vi "ADC SNR_new.vi"(8 "error in (no error)":errorcluster, 9 "Sequence parameters":string[][](array[string])=[["Min limit", "Max limit", "Register sheet file", "Register Sheet"], ["", "", "CC2600.xls", "TX_BLE;Trim"], ["Reg write (addr;value)", "Operating frequency [Hz]", "", ""], ["NA", "2.44G", "", ""]], 10 "Run type":i32, 11 "Method parameters":T4={"Dev"={"Do not disturb DUT"=FALSE, "XOSC"=32000000.0, "Board type"="", "EM"="", "Configure tempboard"=TRUE, "Device specific info"=[], "Generic Object"=refnum}, "Method"={"Run type"=1, "Test name"="Current LPM2 4", "Comment"="", "Results folder"="", "AFC"=enum."Off", "Method name"="Current LPM2 4", "Method results"={"Excel brief report"=FALSE, "Spotfire report"=FALSE, "Starfish report"=FALSE}, "Operator"="", "Reference time"=timestamp(0 s since 1904-01-01), "AFC delay"=0.0, "Initialization"=enum."Enabled", "MD5 Sum"="", "HW addon board"=enum."None", "AFC Regsheet"="", "AFC Regfile"=path "", "dummy"=0.0}, "Inst"={"Instr"={"PS1"={"Name"="", "GPIB address"="", "VISA session"=""}, "PS2"={"Name"="", "GPIB address"="", "VISA session"=""}, "TC1"={"Name"="", "GPIB address"="", "VISA session"=""}, "TC2"={"Name"="", "GPIB address"="", "VISA session"=""}, "SA1"={"Name"="", "GPIB address"="", "VISA session"=""}, "SA2"={"Name"="", "GPIB address"="", "VISA session"=""}, "SG1"={"Name"="", "GPIB address"="", "VISA session"=""}, "SG2"={"Name"="", "GPIB address"="", "VISA session"=""}, "SG3"={"Name"="", "GPIB address"="", "VISA session"=""}, "MI1"={"Name"="", "GPIB address"="", "VISA session"=""}, "MI2"={"Name"="", "GPIB address"="", "VISA session"=""}, "SW SA"={"Name"="", "Controller addr"=""}, "SW SG"={"Name"="", "Controller addr"=""}, "MI3"={"Name"="", "GPIB address"="", "VISA session"=""}}, "Switchbox"={"RF Path"=0, "Cal compensation"=enum."TX", "Switchbox gain mode"="", "State"=enum."TX"}, "Instr to control (i.e. SA1)"="Default", "Intrument info string"=""}, "Sequence parameters"=[["Weight", "Min Limit", "Max Limit", "Register Sheet", "", "", "", "", "", "", "", "", ""], ["Vital", "", "1", "LPM2", "", "", "", "", "", "", "", "", ""], ["Resolution", "Reg write (addr;value)", "Chip mode", "Range", "", "", "", "", "", "", "", "", ""], ["u", "NA", "", "auto", "", "", "", "", "", "", "", "", ""]], "Cond"={"Temp logged"=25.0, "VDD1_PS1_6V"=-999.0, "VDD2_PS1_25V"=-999.0, "VDD4_PS2_25V"=-999.0, "VDD3_PS2_6V"=-999.0}, "Meas config"={"X-axis inner loop index"=32000000, "Y-axis outer loop index"=32000000, "X-axis"=[], "Y-axis"=[], "X-axis array req size"=32000000, "Y-axis array req size"=32000000, "Param description"=[], "Use meas clust for reporting"=FALSE, "Parameter index (page)"=0, "X-axis name"="", "Y-axis name"=""}} {"Cond"."VDD3_PS2_6V" format="%.3f"; "Cond"."VDD4_PS2_25V" format="%.3f"; "Cond"."VDD2_PS1_25V" format="%.3f"; "Cond"."VDD1_PS1_6V" format="%.3f"; "Method"."dummy" format="%.1p"; "Method"."AFC delay" format="%.1p"; "Dev"."XOSC" format="%.3p"}) -> (0 "error out":errorcluster, 1 "End method error":T2, 2 "Short Results":string[](array[string])=["0.00", "0.00", "0.00", "0.00"], 3 "Result summary":string[][](array[string])=[["Critical", "Output Power@2405 MHz", "-3", "4", "dBm"], ["Critical", "Output Power@2410 MHz", "-3", "4", "dBm"]])   [LabVIEW 2019]
doc: "[AutoDocStart]Performs crystal accuracy measurements. Measures the offset from ideal frequency. Primarily used for tuning XOSC capacitors and verifying XOSC trims.\n\nSweeping parameters: operating frequency, OSC override value and VDDR level\n\nResults: Offset frequency in ppm[AutoDocEnd]"
uses:
  User Lib/Utilities/Cluster definitions/DUT VDD1.ctl
  User Lib/Utilities/Cluster definitions/DUT VDD2.ctl
  User Lib/Utilities/Cluster definitions/DUT VDD3.ctl
  User Lib/Utilities/Cluster definitions/DUT VDD4.ctl
  User Lib/Utilities/Cluster definitions/DUT vdd control.ctl
  User Lib/Generic chip methods/Classes/Generic_EM/Chameleon/Loki/Loki.lvclass
  User Lib/Generic chip methods/Classes/Generic_EM/Generic_EM/Generic_EM.lvclass
  User Lib/Utilities/Cluster definitions/Instr clust.ctl
  User Lib/Utilities/Cluster definitions/Method input.ctl
  User Lib/Utilities/Controls/Automatic Frequency Compensation types.ctl
  User Lib/Utilities/Controls/Method Reports.ctl
  User Lib/Utilities/Cluster definitions/End method error cluster.ctl
  User Lib/Utilities/Cluster definitions/Device specific info.ctl
  User Lib/Utilities/Cluster definitions/Method Initialization.ctl
  User Lib/Utilities/Switchbox control/SwitchBox_State._ENUMctl.ctl
  User Lib/Utilities/Controls/HW addon boards.ctl
panel:
  in  "Tab Control":T1(tab)
  out "Dynamic Parameters":T3={"SNR"=nan, "SNRD"=nan, "THD"=nan, "ENOB (SNRD)"=nan, "SFDR"=nan, "ENOB (SNR)"=nan, "Noise Power"=nan, "Signal power"=nan} {"Signal power" format="%.6f"; "Noise Power" format="%.2f"; "ENOB (SNR)" format="%.2f"; "SFDR" format="%.2f"; "ENOB (SNRD)" format="%.2f"; "THD" format="%.2f"; "SNRD" format="%.2f"; "SNR" format="%.2f"}
  out "ADC samples":u32[](array[numeric])
  out "Output Response [All DUTs]":u32[][](array[numeric])
  out "SNR":dbl
  out "Noise Power":dbl
  out "Signal power":dbl
  out "ENOB (SNR)":dbl
  out "detected Throughput":dbl=200065.4236150998
  # "°C"
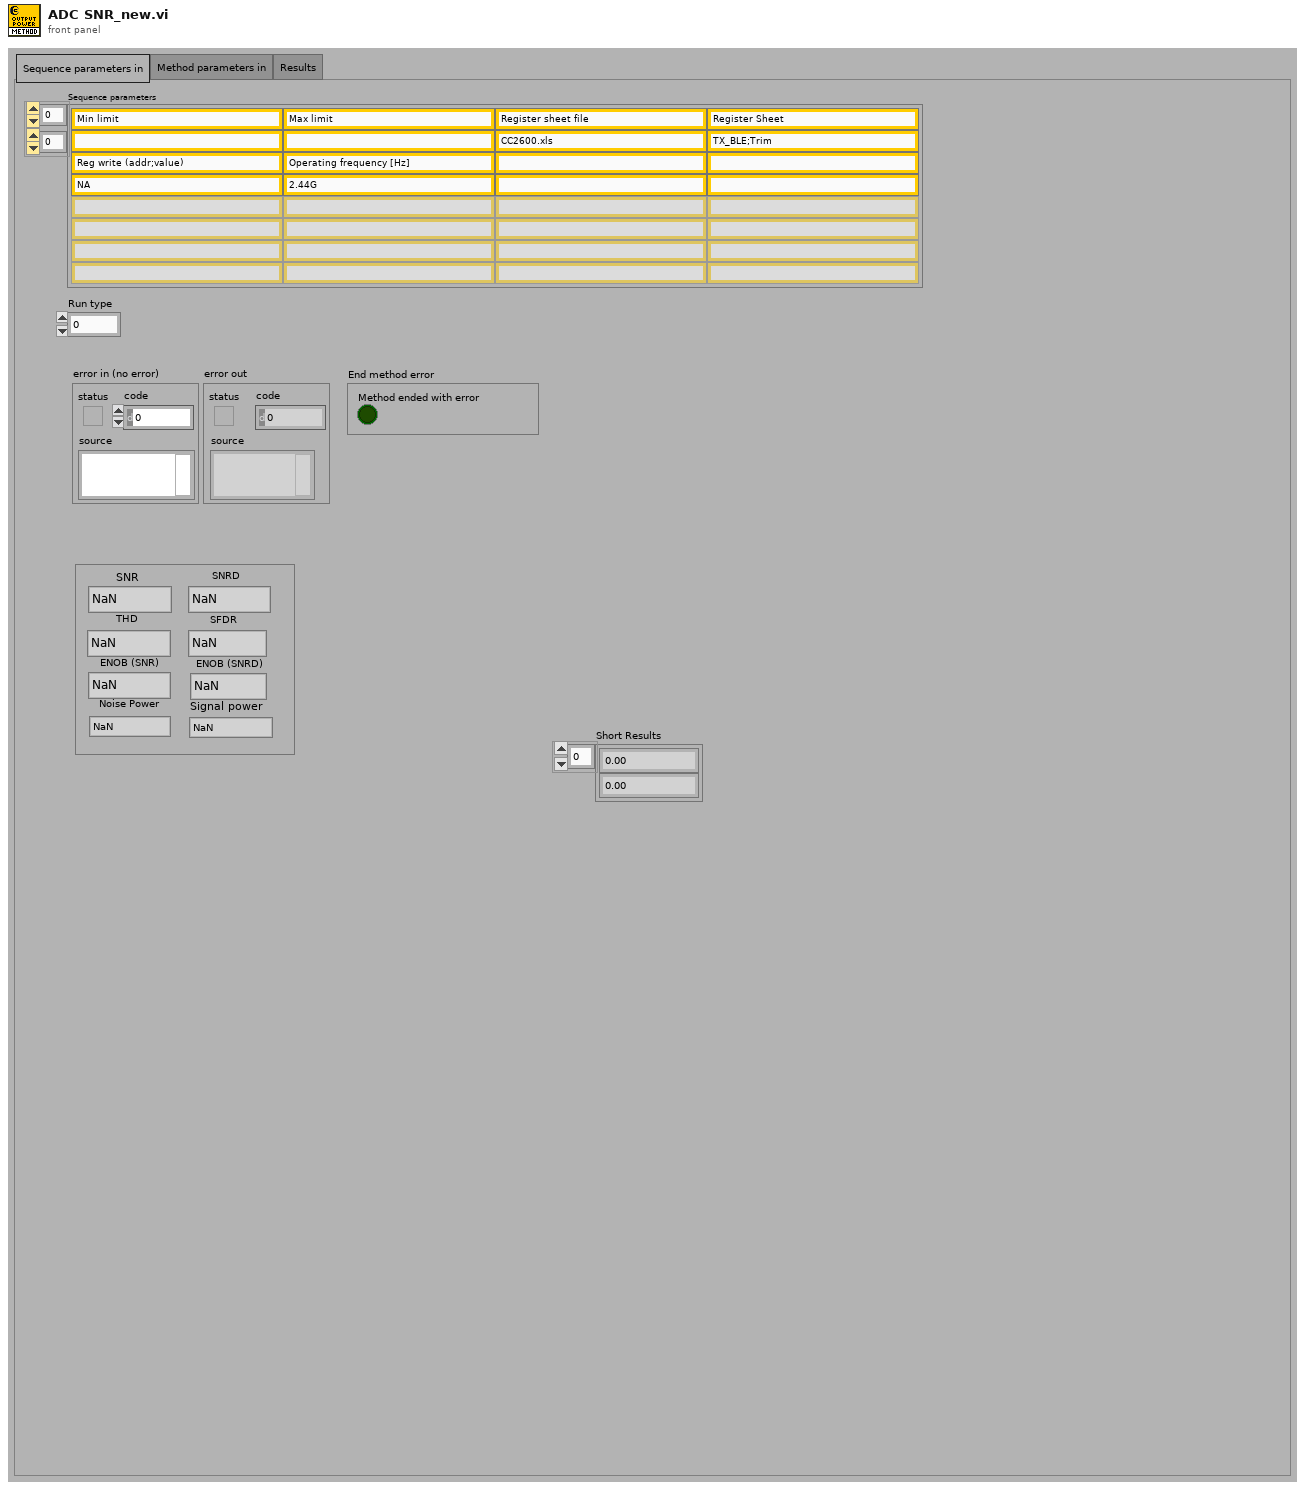
[diagram p1: front panel]
types:
  T1 = enum32{"Sequence parameters in", "Method parameters in", "Results"}
  T2 = typedef "End method error cluster.ctl" = cluster{"Method ended with error":bool}
  T3 = cluster{"SNR":dbl, "SNRD":dbl, "THD":dbl, "ENOB (SNRD)":dbl, "SFDR":dbl, "ENOB (SNR)":dbl, "Noise Power":dbl, "Signal power":dbl}
  T4 = typedef "Method input.ctl" = cluster{"Dev":cluster{"Do not disturb DUT":bool, "XOSC":dbl, "Board type":string, "EM":string, "Configure tempboard":bool, "Device specific info":T5[], "Generic Object":refnum<class>}, "Method":cluster{"Run type":i32, "Test name":string, "Comment":string, "Results folder":string, "AFC":T6, "Method name":string, "Method results":T7, "Operator":string, "Reference time":timestamp, "AFC delay":dbl, "Initialization":T8, "MD5 Sum":string, "HW addon board":T9, "AFC Regsheet":string, "AFC Regfile":path, "dummy":dbl}, "Inst":T10, "Sequence parameters":string[][], "Cond":cluster{"Temp logged":dbl, "VDD1_PS1_6V":dbl, "VDD2_PS1_25V":dbl, "VDD4_PS2_25V":dbl, "VDD3_PS2_6V":dbl}, "Meas config":cluster{"X-axis inner loop index":i32, "Y-axis outer loop index":i32, "X-axis":string[], "Y-axis":string[], "X-axis array req size":i32, "Y-axis array req size":i32, "Param description":string[][], "Use meas clust for reporting":bool, "Parameter index (page)":i32, "X-axis name":string, "Y-axis name":string}}
  T5 = typedef "Device specific info.ctl" = cluster{"EM number":u8, "IP address":string, "Enabled":bool, "Slot no":u8, "RF path":u8, "EM name":string, "Wafer info":string, "AFC frequency ppm":dbl, "Register writes":string[][], "Meas data":string[][][], "Device comment":string}
  T6 = typedef "Automatic Frequency Compensation types.ctl" = enum16{"Off", "Compensate Instrument frequency", "Compensate DUT frequency", "Predictive - Compensate Instrument frequency", "Predictive - Compensate DUT frequency", "Do not skip re-init - Compensate Instrument frequency", "Do not skip re-init - Compensate DUT frequency"}
  T7 = typedef "Method Reports.ctl" = cluster{"Excel brief report":bool, "Spotfire report":bool, "Starfish report":bool}
  T8 = typedef "Method Initialization.ctl" = enum16{"Enabled", "Skip Instr and Device Init", "Enabled with Separate Flash", "Set PS, Device Init and Skip Instr Init", "Skip Device Init"}
  T9 = typedef "HW addon boards.ctl" = enum16{"None", "Current meas 5EM", "Stresstest 10EM"}
  T10 = typedef "Instr clust.ctl" = cluster{"Instr":cluster{"PS1":cluster{"Name":string, "GPIB address":string, "VISA session":refnum<visa-resource-name>}, "PS2":cluster{"Name":string, "GPIB address":string, "VISA session":refnum<visa-resource-name>}, "TC1":cluster{"Name":string, "GPIB address":string, "VISA session":refnum<visa-resource-name>}, "TC2":cluster{"Name":string, "GPIB address":string, "VISA session":refnum<visa-resource-name>}, "SA1":cluster{"Name":string, "GPIB address":string, "VISA session":refnum<visa-resource-name>}, "SA2":cluster{"Name":string, "GPIB address":string, "VISA session":refnum<visa-resource-name>}, "SG1":cluster{"Name":string, "GPIB address":string, "VISA session":refnum<visa-resource-name>}, "SG2":cluster{"Name":string, "GPIB address":string, "VISA session":refnum<visa-resource-name>}, "SG3":cluster{"Name":string, "GPIB address":string, "VISA session":refnum<visa-resource-name>}, "MI1":cluster{"Name":string, "GPIB address":string, "VISA session":refnum<visa-resource-name>}, "MI2":cluster{"Name":string, "GPIB address":string, "VISA session":refnum<visa-resource-name>}, "SW SA":cluster{"Name":string, "Controller addr":string}, "SW SG":cluster{"Name":string, "Controller addr":string}, "MI3":cluster{"Name":string, "GPIB address":string, "VISA session":refnum<visa-resource-name>}}, "Switchbox":cluster{"RF Path":i32, "Cal compensation":enum16{"TX", "RX", "Interferer", "No compensation", "Interferer2"}, "Switchbox gain mode":string, "State":T11}, "Instr to control (i.e. SA1)":string, "Intrument info string":string}
  T11 = typedef "SwitchBox_State._ENUMctl.ctl" = enum16{"TX", "RX", "SP:TX", "SP:RX", "SW:TX", "SW:RX"}
  T12 = typedef "DUT vdd control.ctl" = cluster{"VDD4 config":T13, "VDD3 config":T14, "VDD2 config":T15, "VDD1 config":T16}
  T13 = typedef "DUT VDD4.ctl" = u16
  T14 = typedef "DUT VDD3.ctl" = u16
  T15 = typedef "DUT VDD2.ctl" = u16
  T16 = typedef "DUT VDD1.ctl" = u16
  T17 = cluster{"Path to Save plot":path, "Path to Raw Data plot":path}
  T18 = cluster{"Fundamental Frequency":dbl, "Sampling Frequncy":dbl, "No of Harmonics":u8, "Window":enum16{"None ", "Hanning", "Hamming", "Blackman-Harris", "Exact Blackman", "Blackman", "Flat Top", "4 Term B-Harris ", "7 Term B-Harris"}, "Blackman (fundamental power) bins)":dbl}
  T19 = cluster{"Save INL/DNL Plot(Ramp)":bool, "Save SNR Plot":bool, "Save INL/DNL Plot(Sine)":bool, "Save INL/DNL Raw Data(Ramp)":bool, "Save SNR Raw Data":bool, "Save INL/DNL Raw Data(Sine)":bool, "Save DC Raw data":bool, "Save  Raw Data(Sine)":bool}
  T20 = enum32{"NI Card Settings", "Memory Read Setting", "DC Capture", "ADC Ramp", "ADC Sine", "SNR", "Cap Calibration"}
  T21 = enum32{"Read from Memory", "Read .dat file", "NI Card Capture", "None"}
  T22 = typedef "TFW ResponseData.ctl" = cluster{"errorCode":u32, "executionTime":u32, "processedCmdWord":u32, "responsePar":u32[], "actionCode":u32, "cmdStatus":u16}
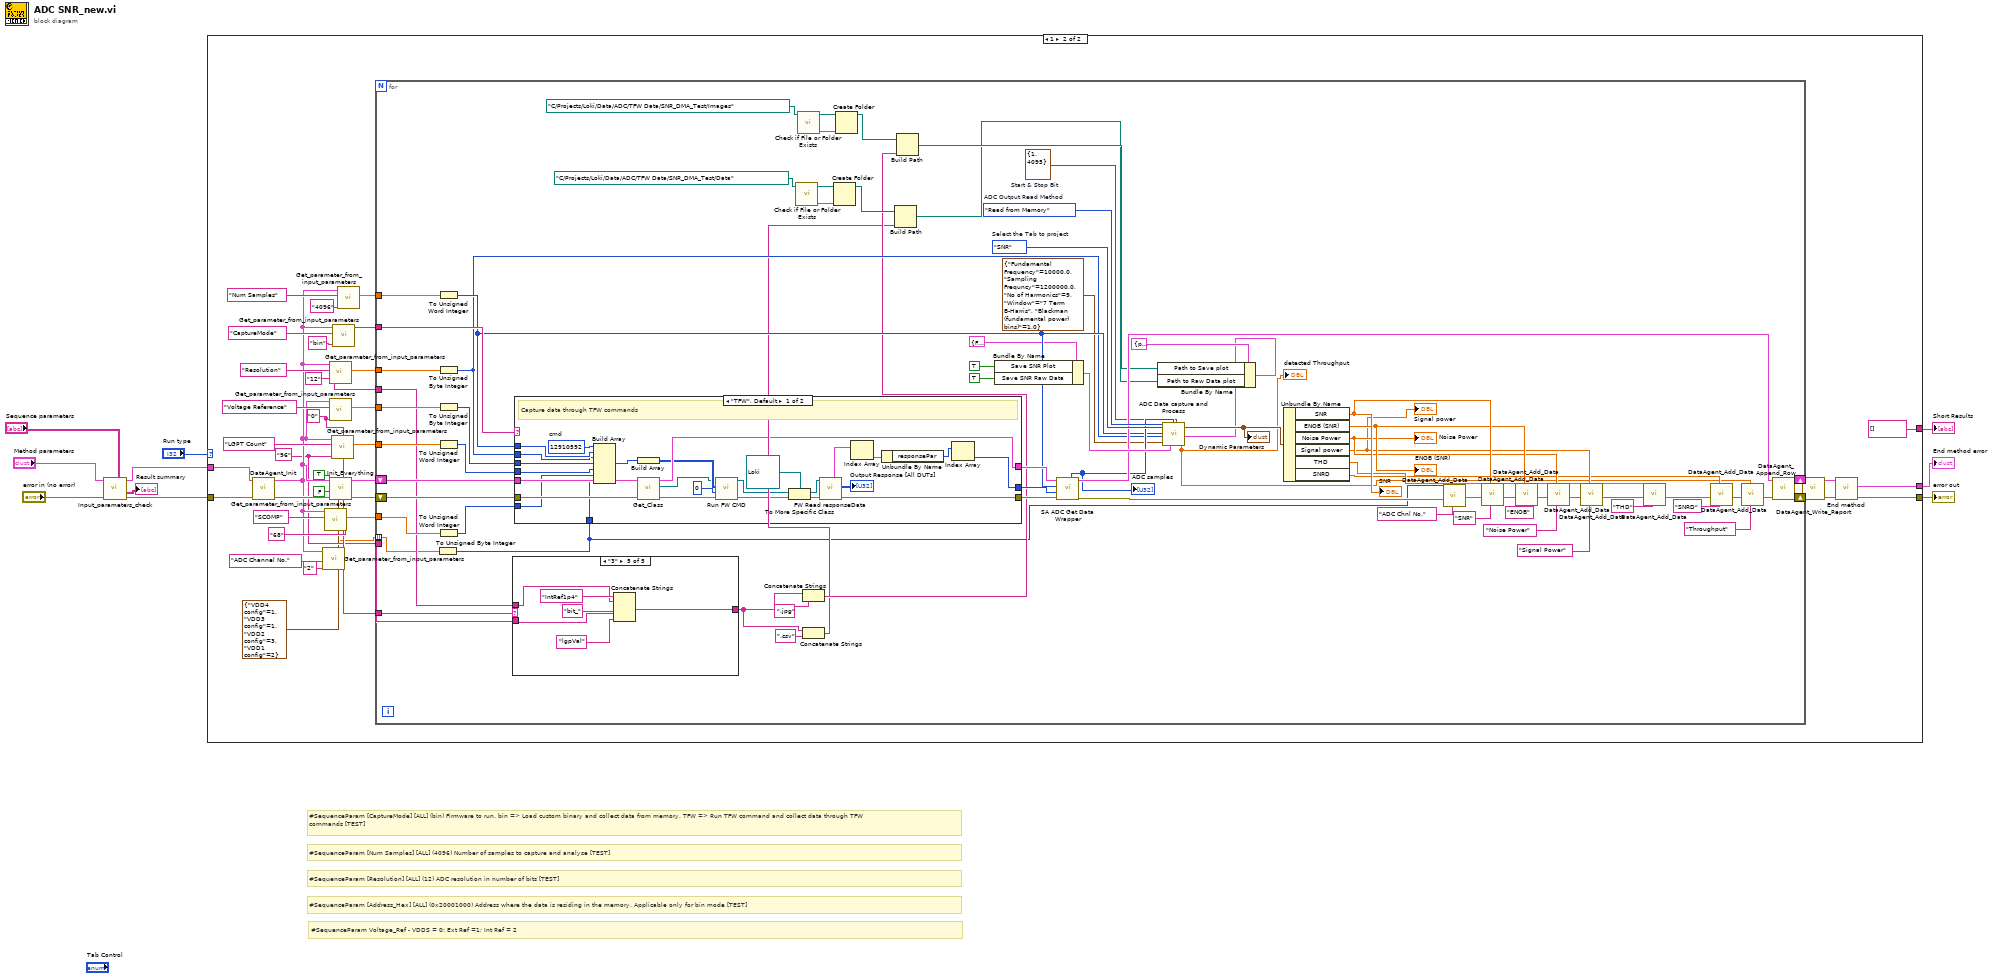
[diagram p0: block diagram]
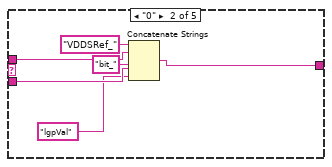
[diagram p4: hidden frame]
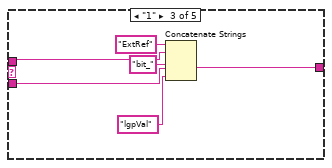
[diagram p5: hidden frame]
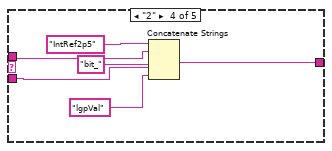
[diagram p6: hidden frame]
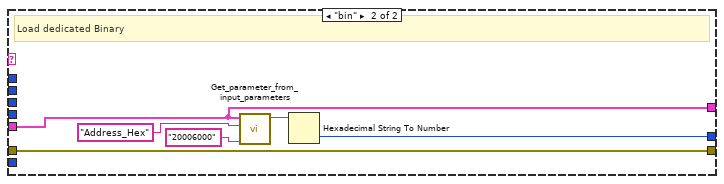
[diagram p7: hidden frame]
diagram:
  # "#SequenceParam Voltage_Ref - VDDS = 0; Ext Ref =1; Int Ref = 2"
  # "#SequenceParam [Num Samples] [ALL] (4096) Number of samples to capture and analyse [TEST]"
  # "#SequenceParam [CaptureMode] [ALL] (bin) Firmware to run. bin => Load custom binary and collect data from memory. TFW => Run TFW command and collect data through TFW commands [TEST]"
  # "#SequenceParam [Address_Hex] [ALL] (0x20001000) Address where the data is residing in the memory. Applicable only for bin mode [TEST]"
  # "#SequenceParam [Resolution] [ALL] (12) ADC resolution in number of bits [TEST]"
  n1 = call "Input_parameters_check.vi"("Sequence parameters"="Sequence parameters", "error in"="error in (no error)", "Method cluster in"="Method parameters") -> ("error out"=w9:errorcluster, "Result summary"=→"Result summary":string[][], "Method cluster out"=w5:T4)  [unwired: 6 in]
  n2 = case shown="1" "Run type" {
    tunnel: w9 -> [w11 w45]
    tunnel: [w11 w48] -> w10
    tunnel: w5 -> [_ w46]
    tunnel: [_ w47] -> w4
    tunnel: [_ string[] []] -> w1
    frame 0, Default {
      # "Run type 0 is only for formatting the result summary"
    }
    frame 1 {
      w15 = "96" ("Default value (used if not specified on Front Panel)")
      w19 = "0" ("Default value (used if not specified on Front Panel)")
      w18 = "12" ("Default value (used if not specified on Front Panel)")
      n3 = call "DataAgent_Init.vi"("error in (no error)"=w45, "Method cluster in"=w46) -> ("error out"=w44:errorcluster, "Method cluster out"=w17:T4)  [unwired: 8 in]
      n4 = call "Get_parameter_from_input_parameters.vi"("Default value (used if not specified on Front Panel)"="2", "Parameter name"="ADC Channel No.", "Method cluster (if input param empty)"=w17) -> ("value as DBL Array"=w13:dbl[])  [unwired: 2 in, 6 out]
      n5 = call "Get_parameter_from_input_parameters.vi"("Default value (used if not specified on Front Panel)"="68", "Parameter name"="SCOMP", "Method cluster (if input param empty)"=w17) -> ("value as DBL"=w20:dbl)  [unwired: 2 in, 6 out]
      n6 = call "Get_parameter_from_input_parameters.vi"("Default value (used if not specified on Front Panel)"=w18, "Parameter name"="Resolution" ("SA_ param name"), "Method cluster (if input param empty)"=w17) -> ("value as DBL"=w26:dbl)  [unwired: 2 in, 6 out]
      n7 = call "Get_parameter_from_input_parameters.vi"("Default value (used if not specified on Front Panel)"=w19, "Parameter name"="Voltage Reference", "Method cluster (if input param empty)"=w17) -> ("value as DBL"=w25:dbl)  [unwired: 2 in, 6 out]
      n8 = call "Init_Everything.vi"("VDD config"=T12 {"VDD4 config"=1, "VDD3 config"=1, "VDD2 config"=3, "VDD1 config"=2}, "error in"=w44, "Support current measurement?"=FALSE, "Override VDD Config"=TRUE, "Method cluster In"=w17) -> ("error out"=w41:errorcluster, "Method cluster out"=w40:T4)  [unwired: 3 in, 2 out]
      n9 = call "Get_parameter_from_input_parameters.vi"("Default value (used if not specified on Front Panel)"=w15, "Parameter name"="LGPT Count", "Method cluster (if input param empty)"=w17) -> ("value as DBL"=w21:dbl)  [unwired: 2 in, 6 out]
      n10 = call "Get_parameter_from_input_parameters.vi"("Default value (used if not specified on Front Panel)"="bin", "Parameter name"="CaptureMode" ("SA_ param name"), "Method cluster (if input param empty)"=w17) -> ("value as String"=w36:string)  [unwired: 2 in, 6 out]
      n11 = call "Get_parameter_from_input_parameters.vi"("Default value (used if not specified on Front Panel)"="4096", "Parameter name"="Num Samples" ("SA_ param name"), "Method cluster (if input param empty)"=w17) -> ("value as DBL"=w34:dbl)  [unwired: 2 in, 6 out]
      n12 = for {
        tunnel: w36 -> [w117]
        tunnel: w34 -> [w111]
        tunnel: w26 -> [w99]
        tunnel: w25 -> [w97]
        tunnel: w21 -> [w95]
        tunnel: w20 -> [w94]
        tunnel: w19 -> [w61]
        tunnel: w18 -> [w60]
        tunnel: w15 -> [w51]
        shift-right: [w108] -> w30
        shift-left: w41 -> [w123]
        shift-right: [w109] -> w31
        shift-left: w40 -> [w122]
        tunnel: w13 -> [w50] mode=indexing
        w100 = cluster{"Start":i32, "Stop":i32} {"Start"=1, "Stop"=4095}  # Start & Stop Bit
        w120 = T20."SNR"  # Select the Tab to project
        w121 = T21."Read from Memory"  # ADC Output Read Method
        n13 = To Unsigned Byte Integer(number=w50) -> (unsigned 8bit integer=w49:u8)
        n14 = To Unsigned Word Integer(number=w111) -> (unsigned 16bit integer=w110:u16)
        n15 = To Unsigned Byte Integer(number=w99) -> (unsigned 8bit integer=w98:u8)
        n16 = To Unsigned Byte Integer(number=w97) -> (unsigned 8bit integer=w96:u8)
        n17 = To Unsigned Word Integer(number=w95) -> (unsigned 16bit integer=w93:u16)
        n18 = To Unsigned Word Integer(number=w94) -> (unsigned 16bit integer=w92:u16)
        n19 = case shown="\"3\"" w61 {
          tunnel: w60 -> [w124 w129 w134 w140 w143]
          tunnel: w51 -> [_ w126 w132 w138 w144]
          tunnel: [w124 w127 w133 w139 w145] -> w58
          frame "False", Default {
          }
          frame "0" {
            n20 = Concatenate Strings("VDDSRef_" ("string"), w129, "bit_" ("string"), w126, "lgpVal" ("string")) -> (w127:string)
          }
          frame "1" {
            n21 = Concatenate Strings("ExtRef" ("string"), w134, "bit_" ("string"), w132, "lgpVal" ("string")) -> (w133:string)
          }
          frame "2" {
            n22 = Concatenate Strings("IntRef2p5" ("string"), w140, "bit_" ("string"), w138, "lgpVal" ("string")) -> (w139:string)
          }
          frame "3" {
            n23 = Concatenate Strings("IntRef1p4" ("string"), w143, "bit_" ("string"), w144, "lgpVal" ("string")) -> (w145:string)
          }
        }
        n24 = case shown="\"TFW\", Default" w117 {
          tunnel: [w174 w175] -> w114
          tunnel: [w167 w180] -> w113
          tunnel: w123 -> [w166 w180]
          tunnel: w122 -> [w173 w175]
          tunnel: [w154 w176] -> w112
          tunnel: w110 -> [w170 _]
          tunnel: w98 -> [w153 _]
          tunnel: w96 -> [w152 _]
          tunnel: w93 -> [w151 _]
          tunnel: w92 -> [w150 _]
          tunnel: w49 -> [w149 _]
          frame "TFW", Default {
            w171 = u32 12910592  # cmd
            # "Capture data through TFW commands"
            n25 = Build Array(w171, w170, w153, w152, w151, w150, w149) -> (w169:u32[])
            n26 = Build Array(w169) -> (w168:u32[][])
            n27 = call "Get_Class.vi"("error in (no error)"=w166, "Method cluster in"=w173) -> ("error out"=w164:errorcluster, "Class Out"=w163:refnum<class "Generic_EM.lvclass">, "Method cluster out"=w174:T4)  [unwired: 6 in, 1 out]
            n28 = call-dynamic "Run FW CMD.vi"("error in (no error)"=w164, "Handler"=u8 0, "cmdBuf"=w168, "Generic_EM in"=w163) -> ("error out"=w159:errorcluster, "Generic_EM out"=w162:refnum<class "Generic_EM.lvclass">)  [unwired: 6 in]
            n29 = To More Specific Class(target class=refnum<class "Loki.lvclass"> refnum ("Loki in"), reference=w162, error in=w159) -> (specific class reference=w160:refnum<class "Loki.lvclass">, error out=w158:errorcluster)
            n30 = call "FW Read responseData.vi"("error in (no error)"=w158, "Loki in"=w160) -> ("error out"=w167:errorcluster, "Output Response [All DUTs]"=→"Output Response [All DUTs]":u32[][], "Response"=w156:T22[])  [unwired: 6 in, 1 out]
            n31 = Index Array(array=w156) -> (element=w157:T22)  [unwired: 1 in]
            n32 = Unbundle By Name(w157) -> ("responsePar"=w155:u32[])
            n33 = Index Array(array=w155) -> (element=w154:u32)  [unwired: 1 in]
          }
          frame "bin" {
            # "Load dedicated Binary"
            n34 = call "Get_parameter_from_input_parameters.vi"("Default value (used if not specified on Front Panel)"="20006000", "Parameter name"="Address_Hex" ("SA_ param name"), "Method cluster (if input param empty)"=w175) -> ("value as String"=w179:string)  [unwired: 2 in, 6 out]
            n35 = Hexadecimal String To Number(string=w179) -> (number=w176:u32)  [unwired: 2 in, 1 out]
          }
        }
        n36 = call <vilib>:"Check if File or Folder Exists.vi"("path"=path "C:/Projects/Loki/Data/ADC/TFW Data/SNR_DMA_Test/Data" ("base path")) -> ("error out"=w66:errorcluster, "dup path"=w65:path)  [unwired: 8 in, 1 out]
        n37 = call <vilib>:"Check if File or Folder Exists.vi"("path"=path "C:/Projects/Loki/Data/ADC/TFW Data/SNR_DMA_Test/Images" ("base path")) -> ("error out"=w71:errorcluster, "dup path"=w70:path)  [unwired: 8 in, 1 out]
        n38 = Concatenate Strings(w58, ".jpg" ("string")) -> (w56:string)
        n39 = Concatenate Strings(w58, ".csv" ("string")) -> (w55:string)
        n40 = Create Folder(path (use dialog)=w65, error in=w66) -> (created path=w63:path)  [unwired: 1 in, 2 out]
        n41 = Create Folder(path (use dialog)=w70, error in=w71) -> (created path=w68:path)  [unwired: 1 in, 2 out]
        n42 = Build Path(base path=w63, name or relative path=w55) -> (appended path=w62:path)
        n43 = Build Path(base path=w68, name or relative path=w56) -> (appended path=w67:path)
        n44 = Bundle By Name(cluster=T19 {"Save INL/DNL Plot(Ramp)"=FALSE, "Save SNR Plot"=FALSE, "Save INL/DNL Plot(Sine)"=FALSE, "Save INL/DNL Raw Data(Ramp)"=FALSE, "Save SNR Raw Data"=FALSE, "Save INL/DNL Raw Data(Sine)"=FALSE, "Save DC Raw data"=FALSE, "Save  Raw Data(Sine)"=FALSE} ("Save data"), "Save SNR Plot"=TRUE, "Save SNR Raw Data"=TRUE) -> (w119:T19)
        n45 = call "SA ADC Get Data Wrapper.vi"("error in"=w113, "Data Address"=w112, "Num Samples"=w110, "Method cluster in"=w114) -> ("error out"=w54:errorcluster, "output cluster"=w116:T4, "ADC samples"=w115:u32[])  [unwired: 2 in, 3 out]
        "ADC samples" <- w115
        n46 = Bundle By Name(cluster=T17 {"Path to Save plot"=path "C:/Projects/Loki/Data/ADC/TFW Data/test.jpg", "Path to Raw Data plot"=path "C:/Projects/Loki/Data/ADC/TFW Data/test.csv"} ("path to save"), "Path to Save plot"=w67, "Path to Raw Data plot"=w62) -> (w90:T17)
        n47 = call "ADC Data capture and Process.vi"("ADC Output Read Method"=w121, "Select the Tab to project"=w120, "No.of samples(SNR)"=w110, "Resolution"=w98, "Inputs for Dyanmic para"=T18 {"Fundamental Frequency"=10000.0, "Sampling Frequncy"=1200000.0, "No of Harmonics"=9, "Window"=enum."7 Term B-Harris", "Blackman (fundamental power) bins)"=1.0}, "Save data"=w119, "Waveform"=w115, "Start & Stop Bit"=w100, "path to save"=w90) -> ("detected Throughput"=w73:dbl, "Dynamic Parameters"=w103:T3)  [unwired: 12 in, 5 out]
        "Dynamic Parameters" <- w103
        "detected Throughput" <- w73
        n48 = Unbundle By Name(w103) -> ("SNR"=w102:dbl, "ENOB (SNR)"=w101:dbl, "Noise Power"=w79:dbl, "Signal power"=w78:dbl, "THD"=w77:dbl, "SNRD"=w76:dbl)
        "SNR" <- w102
        "Noise Power" <- w79
        "Signal power" <- w78
        "ENOB (SNR)" <- w101
        n49 = call "DataAgent_Add_Data.vi"("ColumnName"="ADC Chnl No.", "Data"=w49, "error in (no error)"=w54) -> ("error out"=w53:errorcluster)  [unwired: 8 in]
        n50 = call "DataAgent_Add_Data.vi"("ColumnName"="SNR" ("Default Value"), "Data"=w102, "error in (no error)"=w53) -> ("error out"=w106:errorcluster)  [unwired: 8 in]
        n51 = call "DataAgent_Add_Data.vi"("ColumnName"="ENOB" ("Default Value"), "Data"=w101, "error in (no error)"=w106) -> ("error out"=w87:errorcluster)  [unwired: 8 in]
        n52 = call "DataAgent_Add_Data.vi"("ColumnName"="Noise Power", "Data"=w79, "error in (no error)"=w87) -> ("error out"=w86:errorcluster)  [unwired: 8 in]
        n53 = call "DataAgent_Add_Data.vi"("ColumnName"="Signal Power", "Data"=w78, "error in (no error)"=w86) -> ("error out"=w81:errorcluster)  [unwired: 8 in]
        n54 = call "DataAgent_Add_Data.vi"("ColumnName"="THD", "Data"=w77, "error in (no error)"=w81) -> ("error out"=w80:errorcluster)  [unwired: 8 in]
        n55 = call "DataAgent_Add_Data.vi"("ColumnName"="SNRD", "Data"=w76, "error in (no error)"=w80) -> ("error out"=w74:errorcluster)  [unwired: 8 in]
        n56 = call "DataAgent_Add_Data.vi"("ColumnName"="Throughput", "Data"=w73, "error in (no error)"=w74) -> ("error out"=w75:errorcluster)  [unwired: 8 in]
        n57 = call "DataAgent_Append_Row.vi"("error in (no error)"=w75, "Method cluster in"=w116) -> ("error out"=w108:errorcluster, "Method cluster out"=w109:T4)  [unwired: 8 in]
      }
      n58 = call "DataAgent_Write_Report.vi"("error in (no error)"=w30, "Method cluster in"=w31) -> ("error out"=w43:errorcluster, "Method cluster out"=w42:T4)  [unwired: 8 in]
      n59 = call "End method.vi"("error in"=w43, "Method cluster in"=w42) -> ("error out"=w48:errorcluster, "End method error"=w47:T2)  [unwired: 7 in, 1 out]
    }
  }
  "error out" <- w10
  "End method error" <- w4
  "Short Results" <- w1
